vi "get_config_data.vi"(8 "error in (no error)":errorcluster, 11 "LightSourceAN191011Chameleon in":refnum<class "LightSourceAN191011Chameleon.lvclass">) -> (0 "error out":errorcluster, 2 "config data":T1={"communication settings"={"comm port"="COM4", "data bits"=8, "stop bits"=1, "parity"=enum."none", "baud rate"=enum."19200", "delay before read"=50}, "OME"={"LSID"={"identifier"="", "revision"=0.0}}}, 3 "LightSourceAN191011Chameleon out":refnum<class "LightSourceAN191011Chameleon.lvclass">)   [LabVIEW 2010, in "LightSourceAN191011Chameleon.lvclass"]
uses:
  LightSourceAN191011Chameleon.lvclass
  config_data.ctl
  LightSourceAN191011Chameleon.lvclass/LightSourceAN191011Chameleon.ctl
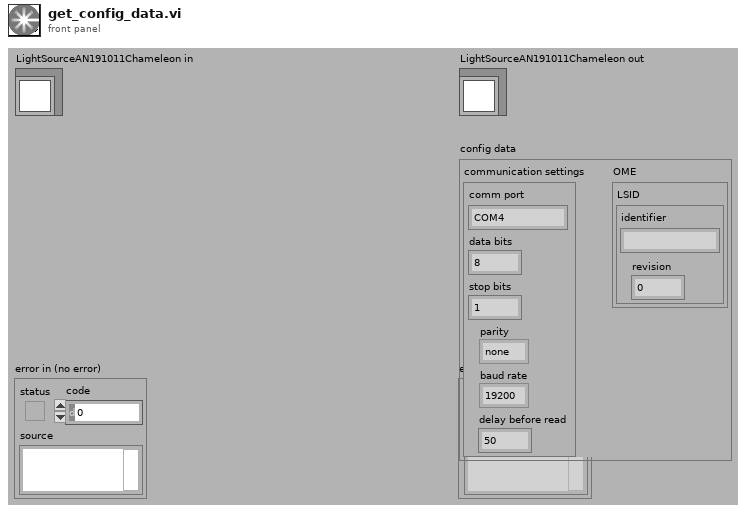
[diagram p1: front panel]
types:
  T1 = typedef "LightSourceAN191011Chameleon.lvclass/config_data.ctl" = cluster{"communication settings":cluster{"comm port":string, "data bits":u8, "stop bits":u8, "parity":enum16{"none", "space", "mark", "even", "odd"}, "baud rate":enum16{"1200", "2400", "4800", "9600", "19200", "38400", "57600"}, "delay before read":u32}, "OME":cluster{"LSID":cluster{"identifier":string, "revision":dbl}}}
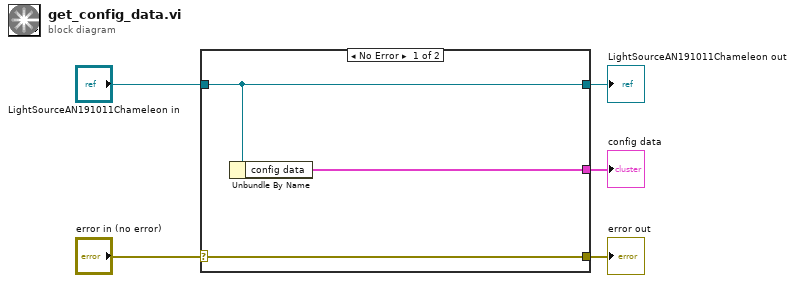
[diagram p0: block diagram]
diagram:
  n1 = case shown="No Error" "error in (no error)" {
    selector: "error in (no error)" -> [w8 w9]
    tunnel: [w8 w9] -> w4
    tunnel: [w7 w10] -> w2
    tunnel: "LightSourceAN191011Chameleon in" -> [w7 w10]
    tunnel: [w6 _] -> w1
    frame No Error {
      n2 = Unbundle By Name(w7) -> ("config data"=w6:T1)
    }
    frame Error {
    }
  }
  "error out" <- w4
  "LightSourceAN191011Chameleon out" <- w2
  "config data" <- w1
